vi "update.vi"(7 "Pressure":dbl, 8 "error in (no error)":errorcluster, 9 "Humidity":dbl, 10 "Temperature":dbl, 11 "CurrentConditionsDisplay.lvclass":refnum<class "CurrentConditionsDisplay.lvclass">) -> (0 "error out":errorcluster, 3 "CurrentConditionsDisplay.lvclass 2":refnum<class "CurrentConditionsDisplay.lvclass">)   [LabVIEW 2020, in "CurrentConditionsDisplay.lvclass"]
uses:
  CurrentConditionsDisplay.lvclass
  CurrentConditionsDisplay.lvclass/CurrentConditionsDisplay.ctl
panel:
  # "Connector Pane"
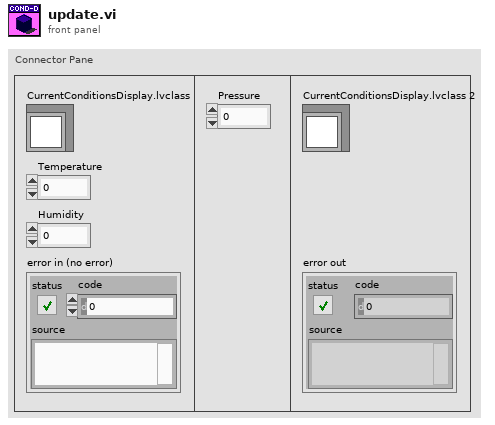
[diagram p1: front panel]
types:
  T1 = typedef "CurrentConditionsDisplay.lvclass/CurrentConditionsData.ctl" = cluster{"Temperature":dbl, "Humidity":dbl}
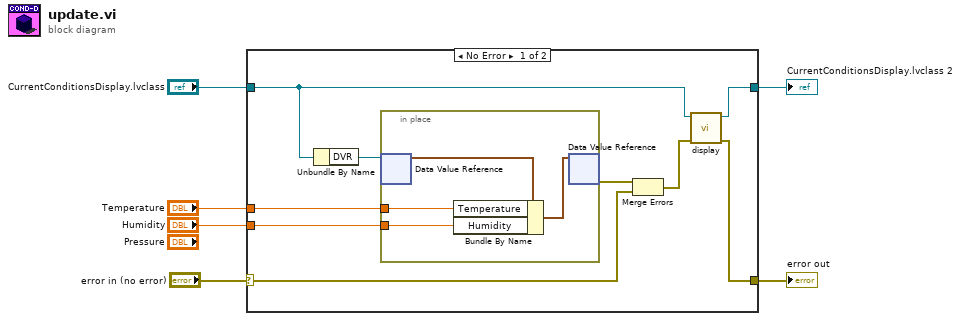
[diagram p0: block diagram]
diagram:
  n1 = case shown="No Error" "error in (no error)" {
    selector: "error in (no error)" -> [w15 w20]
    tunnel: [w14 w20] -> w5
    tunnel: [w13 w21] -> w4
    tunnel: "Temperature" -> [w11 _]
    tunnel: "Humidity" -> [w10 _]
    tunnel: "CurrentConditionsDisplay.lvclass" -> [w9 w21]
    frame No Error {
      n2 = Unbundle By Name(w9) -> ("DVR"=w12:refnum<data-value>)
      n3 = in-place {
        in-place-border: w11 -> [w17]
        in-place-border: w10 -> [w16]
        n4 = in-place-dvr #1(w12) -> (w19:T1)  [unwired: 1 out]
        n5 = Bundle By Name(cluster=w19, "Temperature"=w17, "Humidity"=w16) -> (w18:T1)
        n6 = in-place-dvr #1(w18) -> (w7:errorcluster)  [unwired: 1 out]
      }
      n7 = Merge Errors(w7, w15) -> (w8:errorcluster)
      n8 = call-dynamic "display.vi"("error in (no error)"=w8, "Display"=w9) -> ("error out"=w14:errorcluster, "CurrentConditionsDisplay.lvclass 2"=w13:refnum<class "CurrentConditionsDisplay.lvclass">)  [unwired: 8 in]
    }
    frame Error {
    }
  }
  "CurrentConditionsDisplay.lvclass 2" <- w4
  "error out" <- w5
